vi "DrawScatterPlot.vi"(0 "reference in":refnum<class "LcWebView.lvclass">, 1 "XLabels":string[](array[string]), 2 "ScatterPlot.Dataset":cluster{"x":dbl, "y":dbl}[](array[cluster]), 3 "Scatter.DatasetLabels":string[](array[string]), 5 "Error In":errorcluster, 6 "GenericPlotOptions":T2, 7 "ScatterPlot.PlotColours":u32[](array[numeric]), 8 "ScatterPlotOptions":T1={"xLabel"="", "yLabel"="", "DisplayXLabel"=TRUE, "DisplayYLabel"=TRUE}) -> (14 "reference out":refnum<class "LcWebView.lvclass">, 19 "Error Out":errorcluster)   [LabVIEW 2018, in "LcWebView.lvclass"]
uses:
  LcWebView.lvclass
  ctrls/GenericPlotOption.ctl
  ctrls/LegendPosition.ctl
  ctrls/LinePlotOption.ctl
  cdfa7b6c-348e-4618-b79e-b8b55caa0d01.vi
  <vilib>/JDP Science/JSONtext/Variant to JSON Text.vi
  <vilib>/JDP Science/JSONtext/LVClass Serializer/JSONtext LVClass Serializer.lvclass
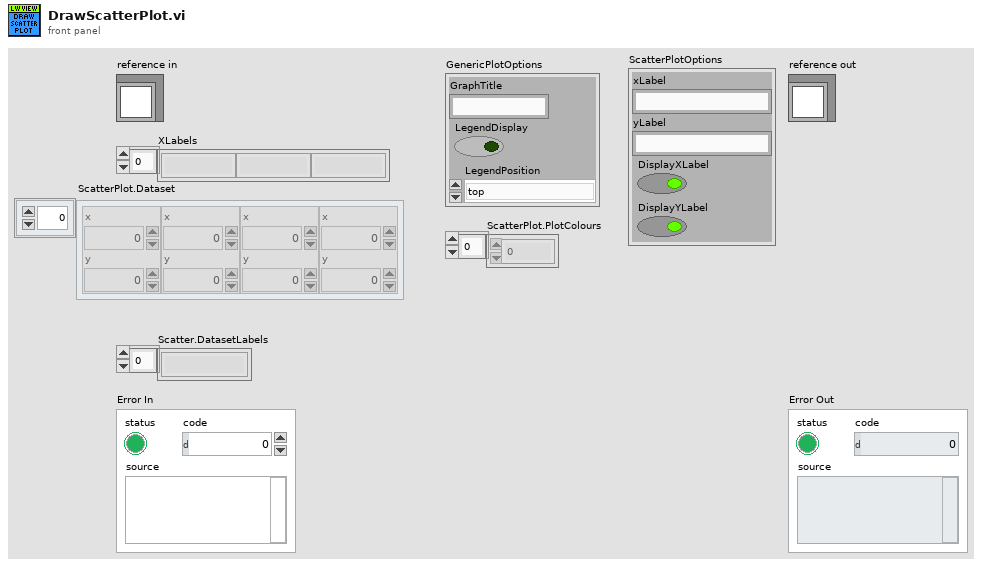
[diagram p1: front panel]
types:
  T1 = typedef "LcWebView.lvclass/LinePlotOption.ctl" = cluster{"xLabel":string, "yLabel":string, "DisplayXLabel":bool, "DisplayYLabel":bool}
  T2 = typedef "LcWebView.lvclass/GenericPlotOption.ctl" = cluster{"GraphTitle":string, "LegendDisplay":bool, "LegendPosition":T3}
  T3 = typedef "LcWebView.lvclass/LegendPosition.ctl" = enum16{"top", "right", "left", "bottom"}
  T4 = cluster{"action":string, "PlotData":string, "GenericPlotOptions":T2, "ScatterPlotOptions":T1}
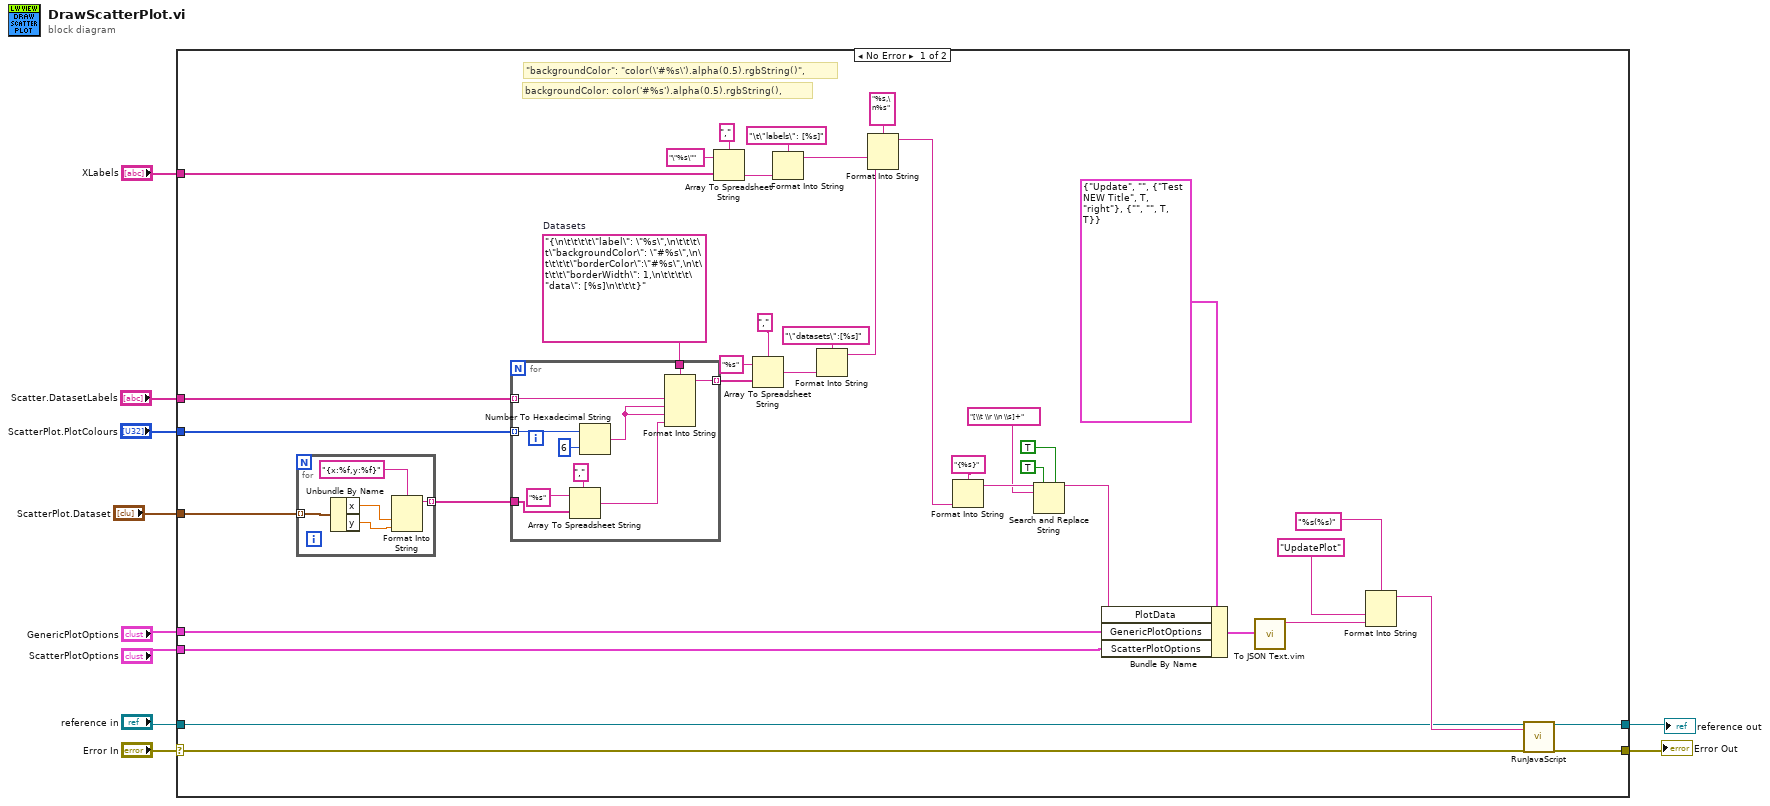
[diagram p0: block diagram]
diagram:
  n1 = case shown="No Error" "Error In" {
    selector: "Error In" -> [w17 w64]
    tunnel: [w18 w64] -> w2
    tunnel: [w19 w63] -> w3
    tunnel: "reference in" -> [w20 w63]
    tunnel: "ScatterPlot.Dataset" -> [w12 _]
    tunnel: "ScatterPlot.PlotColours" -> [w38 _]
    tunnel: "Scatter.DatasetLabels" -> [w37 _]
    tunnel: "XLabels" -> [w36 _]
    tunnel: "GenericPlotOptions" -> [w28 _]
    tunnel: "ScatterPlotOptions" -> [w27 _]
    frame No Error {
      w39 = "{\n\t\t\t\t\"label\": \"%s\",\n\t\t\t\t\"backgroundColor\": \"#%s\",\n\t\t\t\t\"borderColor\":\"#%s\",\n\t\t\t\t\"borderWidth\": 1,\n\t\t\t\t\"data\": [%s]\n\t\t\t}"  # Datasets
      # "\"backgroundColor\": \"color(\\'#%s\\').alpha(0.5).rgbString()\","
      # "backgroundColor: color('#%s').alpha(0.5).rgbString(),"
      n2 = for {
        tunnel: w12 -> [w52] mode=indexing
        tunnel: [w48] -> w11 mode=indexing
        n3 = Unbundle By Name(w52) -> ("x"=w50:dbl, "y"=w49:dbl)
        n4 = Format Into String(format string="{x:%f,y:%f}", w50, w49) -> (resulting string=w48:string)  [unwired: 2 in, 1 out]
      }
      n5 = for {
        tunnel: w38 -> [w59] mode=indexing
        tunnel: w37 -> [w61] mode=indexing
        tunnel: [w60] -> w16 mode=indexing
        tunnel: w39 -> [w62]
        tunnel: w11 -> [w56]
        n6 = Array To Spreadsheet String(delimiter (Tab)="," ("separator"), array=w56, 3:"%s" ("format string")) -> (spreadsheet string=w53:string)
        n7 = Number To Hexadecimal String(1:i16 6 ("width (-)"), 2:w59) -> (0:w58:string)
        n8 = Format Into String(format string=w62, w61, w58, w58, w53) -> (resulting string=w60:string)  [unwired: 2 in, 1 out]
      }
      n9 = Array To Spreadsheet String(delimiter (Tab)=",", array=w36, 3:"\"%s\"" ("format string")) -> (spreadsheet string=w43:string)
      n10 = Array To Spreadsheet String(delimiter (Tab)="," ("separator"), array=w16, 3:"%s" ("format string")) -> (spreadsheet string=w13:string)
      n11 = Format Into String(format string="\t\"labels\": [%s]", w43) -> (resulting string=w46:string)  [unwired: 2 in, 1 out]
      n12 = Format Into String(format string="\"datasets\":[%s]", w13) -> (resulting string=w41:string)  [unwired: 2 in, 1 out]
      n13 = Format Into String(format string="%s,\n%s", w46, w41) -> (resulting string=w34:string)  [unwired: 2 in, 1 out]
      n14 = Format Into String(format string="{%s}", w34) -> (resulting string=w33:string)  [unwired: 2 in, 1 out]
      n15 = Search and Replace String(replace all?=TRUE ("replace all? (F)"), multiline?=TRUE ("multiline? (F)"), input string=w33, search string="[\\t \\r \\n \\s]+") -> (result string=w32:string)  [unwired: 4 in, 3 out]
      n16 = Bundle By Name(cluster=T4 {"action"="Update", "PlotData"="", "GenericPlotOptions"={"GraphTitle"="Test NEW Title", "LegendDisplay"=TRUE, "LegendPosition"=enum."right"}, "ScatterPlotOptions"={"xLabel"="", "yLabel"="", "DisplayXLabel"=TRUE, "DisplayYLabel"=TRUE}}, "PlotData"=w32, "GenericPlotOptions"=w28, "ScatterPlotOptions"=w27) -> (w25:T4)
      n17 = call "To JSON Text.vim"("Anything"=w25) -> ("<JSON>"=w22:string)  [unwired: 9 in, 1 out]
      n18 = Format Into String(format string="%s(%s)", "UpdatePlot" ("input 1"), w22) -> (resulting string=w21:string)  [unwired: 2 in, 1 out]
      n19 = call-dynamic "RunJavaScript.vi"("reference in"=w20, "Java Script Function"=w21, "Error In"=w17) -> ("reference out"=w19:refnum<class "LcWebView.lvclass">, "Error Out"=w18:errorcluster)  [unwired: 13 in, 2 out]
    }
    frame Error {
    }
  }
  "Error Out" <- w2
  "reference out" <- w3
